vi "解析协议.vi"(4 "输入":string) -> (0 "解析成功?":bool, 1 "输出":T1)   [LabVIEW 2017]
panel:
  out "输出":string
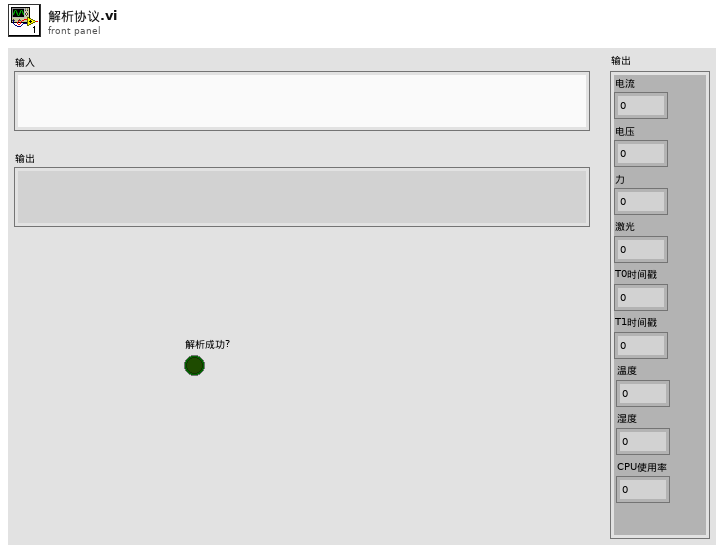
[diagram p1: front panel]
types:
  T1 = cluster{"电流":dbl, "电压":dbl, "力":dbl, "激光":dbl, "T0时间戳":dbl, "T1时间戳":dbl, "温度":dbl, "湿度":dbl, "CPU使用率":dbl}
  T2 = cluster{dbl, dbl, dbl, dbl, dbl, dbl, dbl, dbl, dbl}
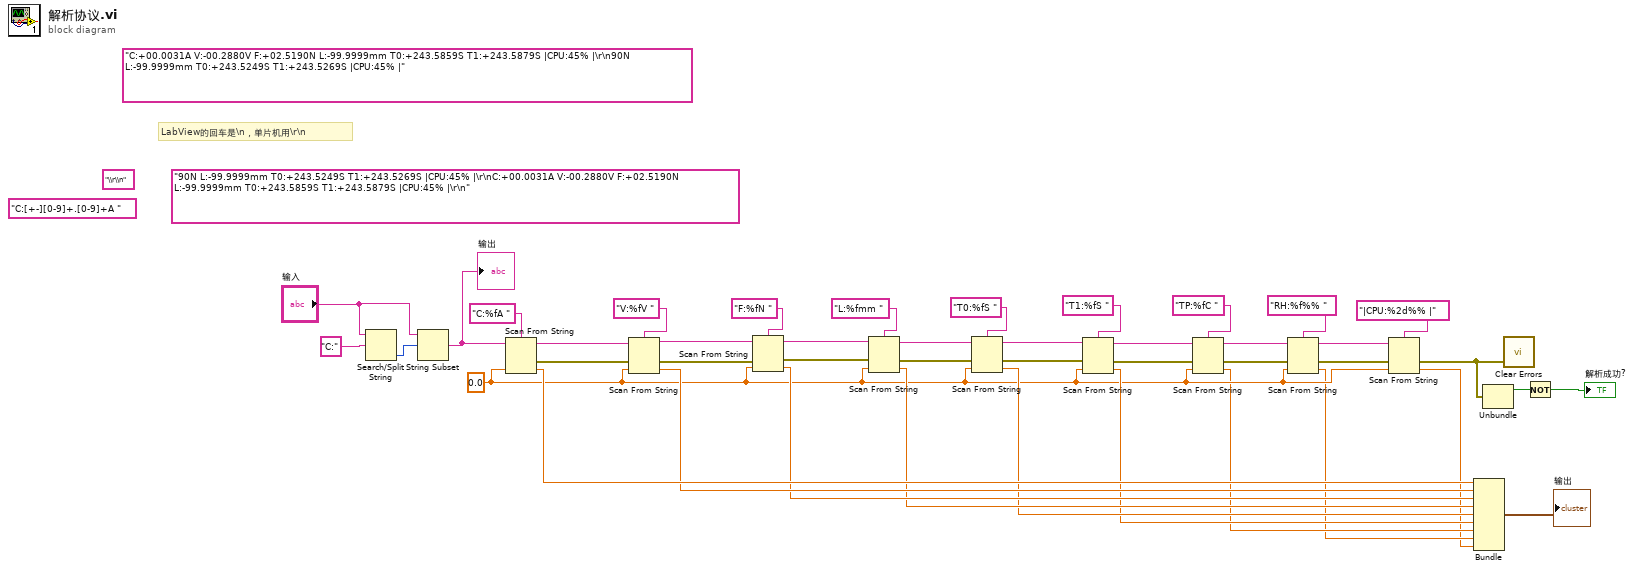
[diagram p0: block diagram]
diagram:
  (unwired) "C:+00.0031A V:-00.2880V F:+02.5190N L:-99.9999mm T0:+243.5859S T1:+243.5879S |CPU:45% |\r\n90N L:-99.9999mm T0:+243.5249S T1:+243.5269S |CPU:45% |"
  (unwired) "\\r\\n"
  w7 = 0.0
  (unwired) "C:[+-][0-9]+.[0-9]+A "
  (unwired) "90N L:-99.9999mm T0:+243.5249S T1:+243.5269S |CPU:45% |\r\nC:+00.0031A V:-00.2880V F:+02.5190N L:-99.9999mm T0:+243.5859S T1:+243.5879S |CPU:45% |\r\n"
  # "LabView的回车是\\n，单片机用\\r\\n"
  n1 = Search/Split String(string="输入", search string/char (-)="C:") -> (offset of match=w18:i32)  [unwired: 1 in, 2 out]
  n2 = String Subset(string="输入", offset (0)=w18) -> (substring=w14:string)  [unwired: 1 in]
  "输出" <- w14
  n3 = Scan From String(format string="C:%fA ", input string=w14, default 1=w7) -> (remaining string=w42:string, error out=w37:errorcluster, output 1=w25:dbl)  [unwired: 2 in, 1 out]
  n4 = Scan From String(format string="V:%fV ", input string=w42, error in=w37, default 1=w7) -> (remaining string=w40:string, error out=w36:errorcluster, output 1=w24:dbl)  [unwired: 1 in, 1 out]
  n5 = Scan From String(format string="F:%fN ", input string=w40, error in=w36, default 1=w7) -> (remaining string=w34:string, error out=w35:errorcluster, output 1=w23:dbl)  [unwired: 1 in, 1 out]
  n6 = Scan From String(format string="L:%fmm ", input string=w34, error in=w35, default 1=w7) -> (remaining string=w32:string, error out=w31:errorcluster, output 1=w22:dbl)  [unwired: 1 in, 1 out]
  n7 = Scan From String(format string="T0:%fS ", input string=w32, error in=w31, default 1=w7) -> (remaining string=w30:string, error out=w27:errorcluster, output 1=w21:dbl)  [unwired: 1 in, 1 out]
  n8 = Scan From String(format string="T1:%fS ", input string=w30, error in=w27, default 1=w7) -> (remaining string=w10:string, error out=w2:errorcluster, output 1=w20:dbl)  [unwired: 1 in, 1 out]
  n9 = Scan From String(format string="TP:%fC ", input string=w10, error in=w2, default 1=w7) -> (remaining string=w9:string, error out=w1:errorcluster, output 1=w6:dbl)  [unwired: 1 in, 1 out]
  n10 = Scan From String(format string="RH:%f%% ", input string=w9, error in=w1, default 1=w7) -> (remaining string=w8:string, error out=w12:errorcluster, output 1=w5:dbl)  [unwired: 1 in, 1 out]
  n11 = Scan From String(format string="|CPU:%2d%% |", input string=w8, error in=w12, default 1=w7) -> (error out=w26:errorcluster, output 1=w4:dbl)  [unwired: 1 in, 2 out]
  n12 = Bundle(w25, w24, w23, w22, w21, w20, w6, w5, w4) -> (→"输出":T2)  [unwired: 1 in]
  n13 = Unbundle(w26) -> ("status"=w16:bool)  [unwired: 2 out]
  n14 = call <vilib>:"Clear Errors.vi"("error in (no error)"=w26) -> ()  [unwired: 5 in, 2 out]
  n15 = Not(x=w16) -> (.not. x?=→"解析成功?":bool)
